vi "sub_psk_demod.vi"(8 "index map":i32[](array[numeric]), 9 "symbol map":cdb[](array[numeric]), 11 "symbol":cdb[](array[numeric])) -> (3 "bitstream":i16[](array[numeric]))   [LabVIEW 2014]
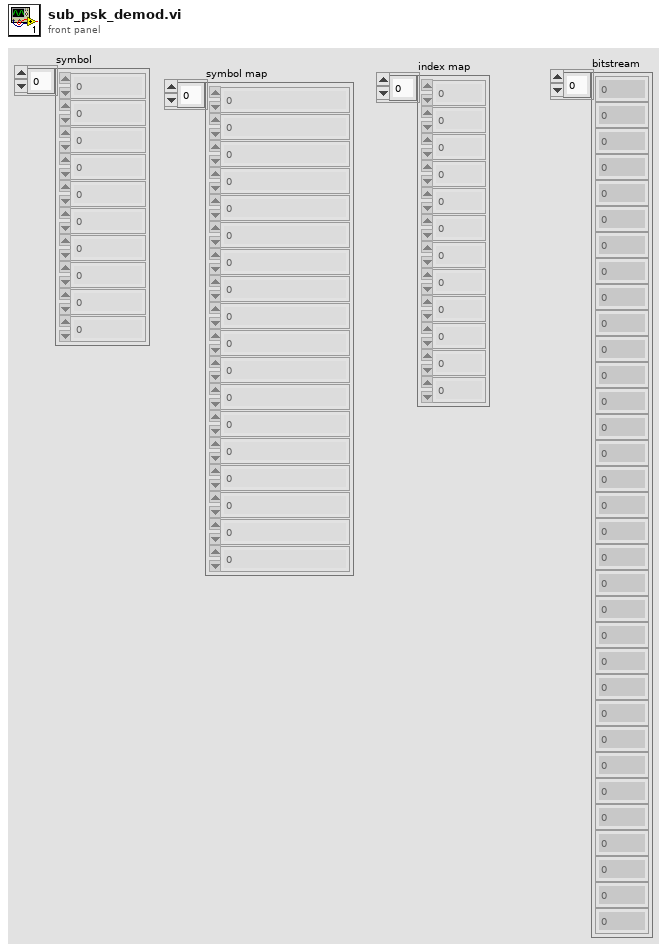
[diagram p1: front panel]
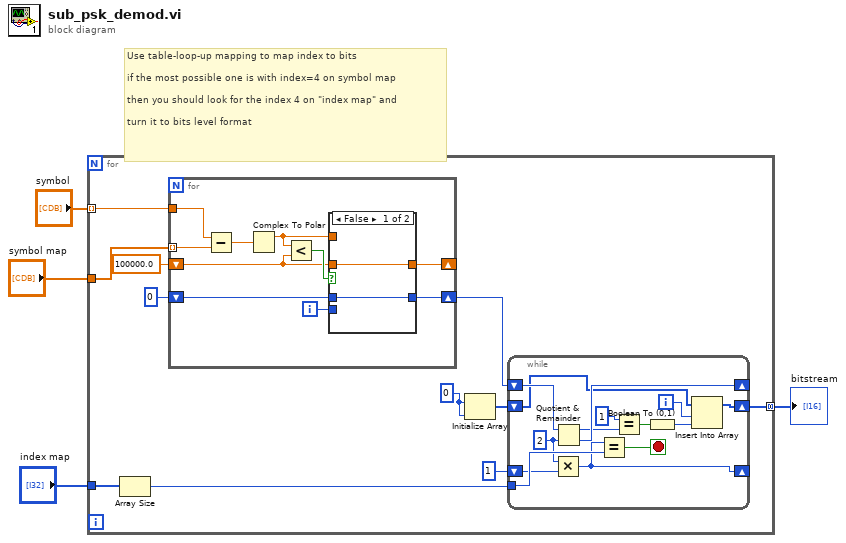
[diagram p0: block diagram]
diagram:
  # "Use table-loop-up mapping to map index to bits\n\nif the most possible one is with index=4 on symbol map\n\nthen you should look for the index 4 on \"index map\" and\n\nturn it to bits level format"
  n1 = for {
    tunnel: "symbol" -> [w14] mode=indexing
    tunnel: "symbol map" -> [w15]
    tunnel: "index map" -> [w11]
    tunnel: [w6] -> w1 mode=concatenating
    w8 = 0
    n2 = Array Size(array=w11) -> (size(s)=w10:i32)
    n3 = for {
      tunnel: w15 -> [w38] mode=indexing
      tunnel: w14 -> [w39]
      shift-right: [w30] -> _
      shift-left: 100000.0 -> [w31]
      shift-right: [w33] -> w5
      shift-left: 0 -> [w35]
      i -> [w36]
      n4 = Subtract(x=w39, y=w38) -> (x-y=w37:cdb)
      n5 = Complex To Polar(r * e^(i*theta)=w37) -> (r=w32:dbl)  [unwired: 1 out]
      n6 = Less?(x=w32, y=w31) -> (x < y?=w34:bool)
      n7 = case shown="False" w34 {
        tunnel: w36 -> [_ w43]
        tunnel: w35 -> [w40 _]
        tunnel: [w40 w43] -> w33
        tunnel: w32 -> [_ w42]
        tunnel: w31 -> [w41 _]
        tunnel: [w41 w42] -> w30
        frame False {
        }
        frame True {
        }
      }
    }
    n8 = Initialize Array(w8, w8) -> (w7:i32[])
    n9 = while {
      tunnel: w10 -> [w29]
      shift-right: [w17] -> _
      shift-left: 1 -> [w28]
      shift-right: [w18] -> w6
      shift-left: w7 -> [w20]
      shift-right: [w24] -> _
      shift-left: w5 -> [w26]
      i -> [w16]
      stop <- w27 stop-if-true
      w25 = 2
      n10 = Multiply(x=w25, y=w28) -> (x*y=w17:i32)
      n11 = Quotient & Remainder(x=w26, y=w25) -> (x-y*floor(x/y)=w22:i32, floor(x/y)=w24:i32)
      n12 = Equal?(x=w17, y=w29) -> (x = y?=w27:bool)
      n13 = Equal?(x=1, y=w22) -> (x = y?=w21:bool)
      n14 = Boolean To (0,1)(Boolean=w21) -> (0, 1=w19:i16)
      n15 = Insert Into Array(array=w20, index=w16, new element=w19) -> (w18:i32[])
    }
  }
  "bitstream" <- w1
